vi "机台号设置.vi"() -> (2 "确定":bool)   [LabVIEW 2020]
uses:
  Global.vi
  <vilib>/Utility/config.llb/Write Key (String).vi
  <vilib>/Utility/config.llb/NI_LVConfig.lvlib
panel:
  out "error out":errorcluster caption="错误输出"
  in  "error in":errorcluster caption="错误输入（无错误）"
  in  "机台号":string="#01"
  in  "取消":bool
  in  "确定":bool
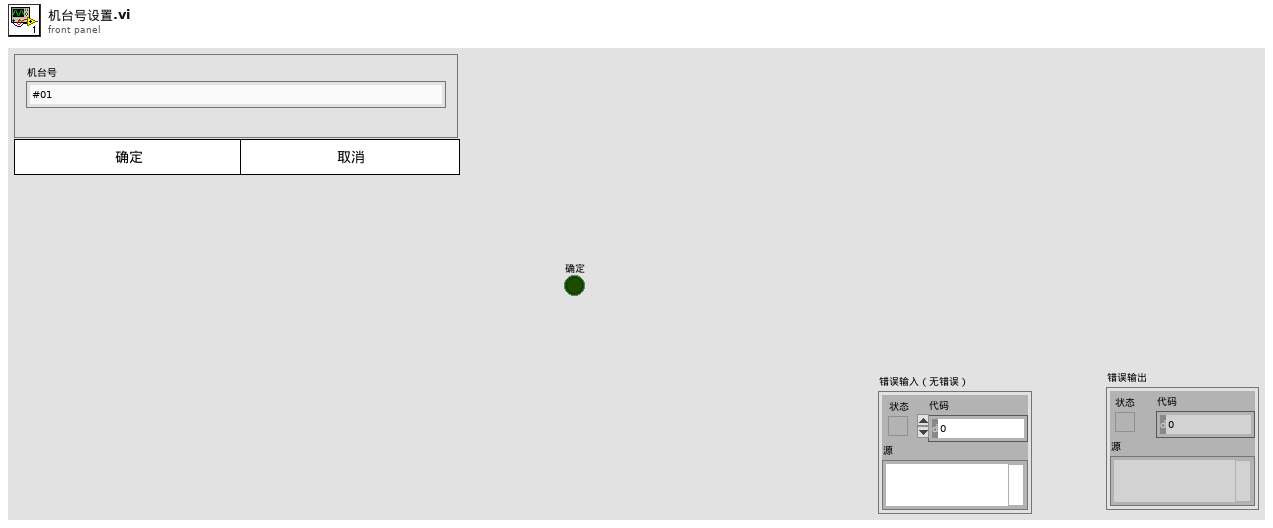
[diagram p1: front panel]
types:
  T1 = typedef "NI_LVConfig.lvlib/Config Data RefNum.ctl" = refnum<k1>
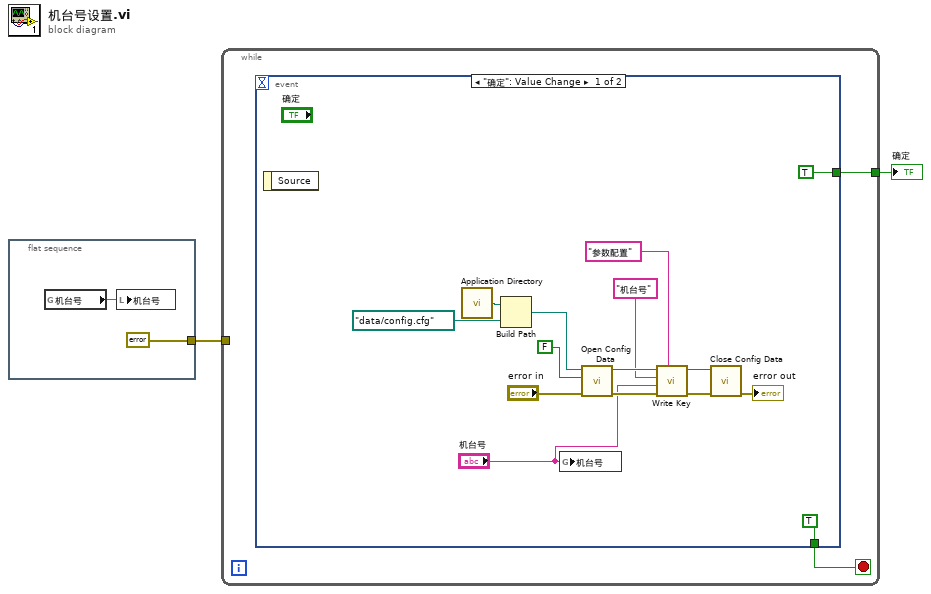
[diagram p0: block diagram]
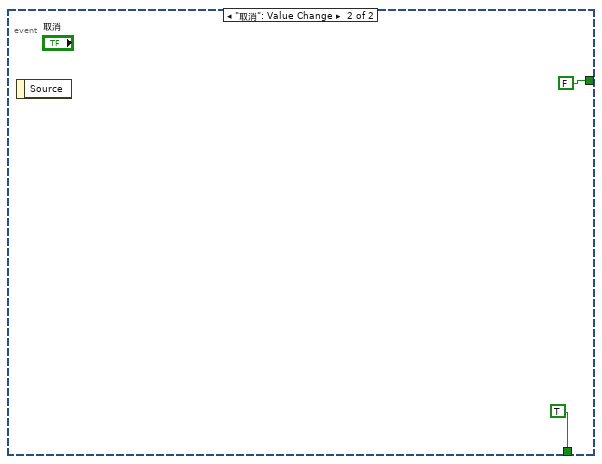
[diagram p2: hidden frame]
diagram:
  n1 = flat-sequence {
    tunnel: [errorcluster {"status"=FALSE, "code"=0, "source"=""} ("错误常量")] -> w1
    frame #0 {
      n2 = global read "Global.vi" "机台号"() -> (w3:string)
      n3 = local write "机台号"(w3) -> ()
    }
  }
  n4 = while {
    tunnel: [w5] -> w2
    tunnel: w1 -> [_]
    stop <- w6 stop-if-true
    n5 = event shown="[0] \"确定\": Value Change" {
      selector: _ -> [_ _]
      dyn-events: _ -> [_ _]
      timeout: _ -> [_ _]
      tunnel: [TRUE TRUE] -> w6
      tunnel: [TRUE FALSE] -> w5
      event "确定": Value Change {
        n6 = event-data() -> ()  [unwired: 1 in, 1 out]
        n7 = call <vilib>:"Application Directory.vi"() -> ("Application Directory"=w12:path)
        n8 = Build Path(base path=w12, name or relative path=path "data/config.cfg") -> (appended path=w13:path)
        n9 = global write "Global.vi" "机台号"("机台号") -> ()
        n10 = call <vilib>:"Open Config Data.vi"("error in (no error)"="error in", "create file if necessary (T)"=FALSE, "configuration file path"=w13) -> ("error out"=w16:errorcluster, "refnum"=w15:T1)  [unwired: 6 in, 1 out]
        n11 = call-poly <vilib>:"Write Key.vi"("section"="参数配置", "error in (no error)"=w16, "value"="机台号", "key"="机台号" ("section"), "refnum"=w15) -> ("error out"=w18:errorcluster, "refnum out"=w17:T1)  [unwired: 4 in, 1 out]
        n12 = call <vilib>:"Close Config Data.vi"("error in (no error)"=w18, "refnum"=w17) -> ("error out"=→"error out":errorcluster)  [unwired: 8 in, 1 out]
      }
      event "取消": Value Change {
        n13 = event-data() -> ()  [unwired: 1 in, 1 out]
      }
    }
  }
  "确定" <- w2
